vi "Get DDG Optical Width Enabled.vi"(8 "error in (no error)":errorcluster, 11 "puiEnabled":u32) -> (0 "error out":errorcluster, 2 "function return":u32, 3 "puiEnabled out":u32)   [LabVIEW 2014, in "atmcd32d.lvlib"]
doc: "unsigned int WINAPI GetDDGOpticalWidthEnabled(at_u32 * puiEnabled);"
uses:
  atmcd32d.lvlib
  atmcd32d.dll
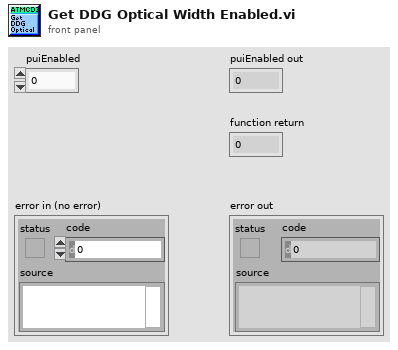
[diagram p1: front panel]
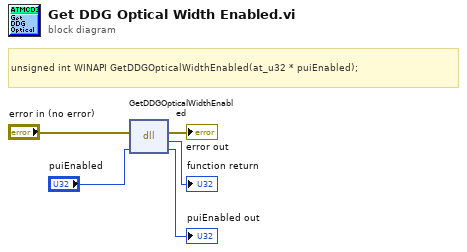
[diagram p0: block diagram]
diagram:
  # "unsigned int WINAPI GetDDGOpticalWidthEnabled(at_u32 * puiEnabled);"
  n1 = dll-call lib="C:/Users/Bakir/Documents/Lambda2-Testing/lib/Andorlib/atmcd32d.*" fn="GetDDGOpticalWidthEnabled"(error in="error in (no error)", "puiEnabled"="puiEnabled") -> (error out=→"error out":errorcluster, →"function return":u32, "puiEnabled"=→"puiEnabled out":u32)  [unwired: 2 in, 1 out]
